vi "setMenuItemTag.vi"(8 "error in (no error)":errorcluster, 10 "Menu Item Tag":string, 11 "Handle Menu Actions in":refnum<class "Handle Menu Actions.lvclass">) -> (0 "error out":errorcluster, 3 "Handle Menu Actions out":refnum<class "Handle Menu Actions.lvclass">)   [LabVIEW 2020, in "Handle Menu Actions.lvclass"]
uses:
  Handle Menu Actions.lvclass
  Handle Menu Actions.lvclass/Handle Menu Actions.ctl
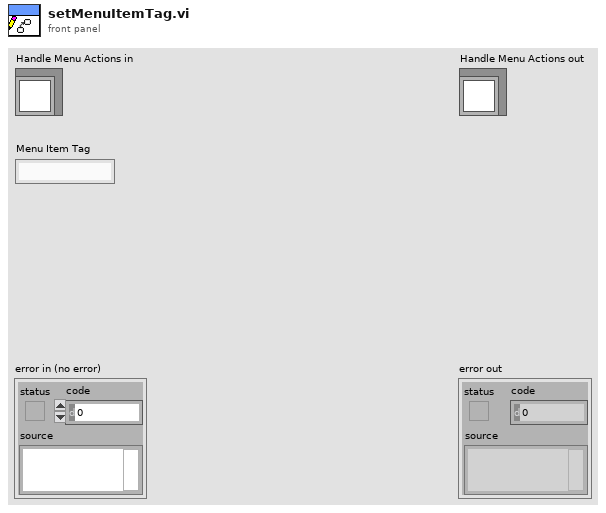
[diagram p1: front panel]
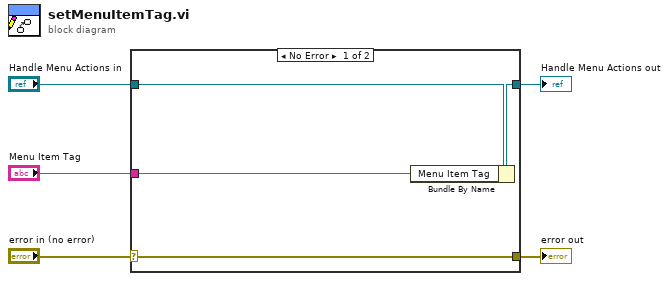
[diagram p0: block diagram]
diagram:
  n1 = case shown="No Error" "error in (no error)" {
    selector: "error in (no error)" -> [w9 w10]
    tunnel: [w9 w10] -> w4
    tunnel: [w7 w11] -> w2
    tunnel: "Handle Menu Actions in" -> [w8 w11]
    tunnel: "Menu Item Tag" -> [w6 _]
    frame No Error {
      n2 = Bundle By Name(cluster=w8, "Menu Item Tag"=w6) -> (w7:refnum<class "Handle Menu Actions.lvclass">)
    }
    frame Error {
    }
  }
  "error out" <- w4
  "Handle Menu Actions out" <- w2
